vi "Get Value.vi"(8 "error in (no error)":errorcluster, 11 "DA Child B in":refnum<class "DA Child B.lvclass">) -> (0 "error out":errorcluster, 2 "Value":string, 3 "DA Child B out":refnum<class "DA Child B.lvclass">)   [LabVIEW 2014, in "Display As.lvlib" / "DA Child B.lvclass"]
uses:
  DA Child B.lvclass
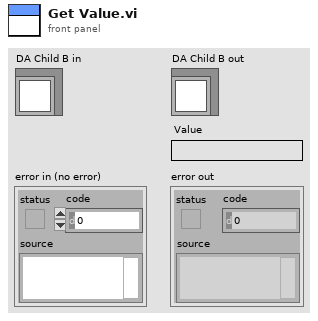
[diagram p1: front panel]
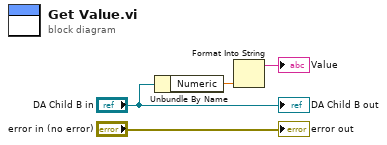
[diagram p0: block diagram]
diagram:
  n1 = Unbundle By Name("DA Child B in") -> ("Numeric"=w2:dbl)
  n2 = Format Into String(w2) -> (resulting string=→"Value":string)  [unwired: 3 in, 1 out]
  "error out" <- "error in (no error)"
  "DA Child B out" <- "DA Child B in"
